vi "ReadData.vi"() -> (0 "Data":string[][](array[string]))   [LabVIEW 2016]
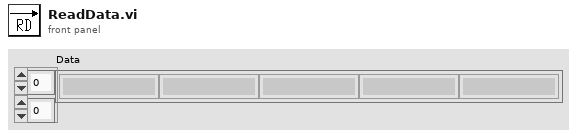
[diagram p1: front panel]
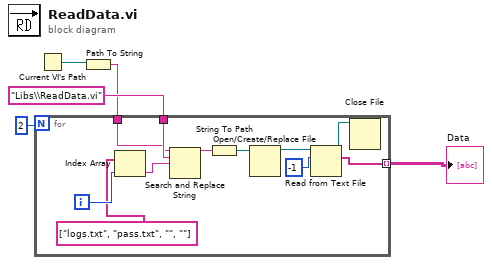
[diagram p0: block diagram]
diagram:
  n1 = Current VI's Path() -> (path=w5:path)
  n2 = Path To String(path=w5) -> (string=w1:string)
  n3 = for {
    N: 2 -> [_]
    tunnel: "Libs\\ReadData.vi" -> [w15]
    tunnel: w1 -> [w14]
    tunnel: [w9] -> w2 mode=indexing
    i -> [w12]
    n4 = Index Array(array=string[] ["logs.txt", "pass.txt", "", ""], index=w12) -> (element=w6:string)
    n5 = Search and Replace String(input string=w14, search string=w15, replace string=w6) -> (result string=w8:string)  [unwired: 5 in, 3 out]
    n6 = String To Path(string=w8) -> (path=w16:path)
    n7 = Open/Create/Replace File(file path (use dialog)=w16) -> (refnum out=w13:refnum<file>)  [unwired: 5 in, 2 out]
    n8 = Read from Text File(file (use dialog)=w13, count=-1) -> (refnum out=w10:refnum<file>, text=w9:string[])  [unwired: 2 in, 2 out]
    n9 = Close File(refnum=w10) -> ()  [unwired: 1 in, 2 out]
  }
  "Data" <- w2
